vi "Get WorksheetPart.vi"(8 "error in":errorcluster, 10 "Sheet Name":string, 11 "SpreadsheetDocument in":refnum<k24>) -> (0 "error out":errorcluster, 2 "WorksheetPart":refnum<k24>, 3 "SpreadsheetDocument out":refnum<k24>)   [LabVIEW 2021, in "Open Xml.lvlib"]
uses:
  Open Xml.lvlib
  D:/git/Open-Xml-LabVIEW/dll/DocumentFormat.OpenXml.dll
  dll/DocumentFormat.OpenXml.dll
  D:/git/Open-Xml-LabVIEW/dll/DocumentFormat.OpenXml.Framework.dll
  dll/DocumentFormat.OpenXml.Framework.dll
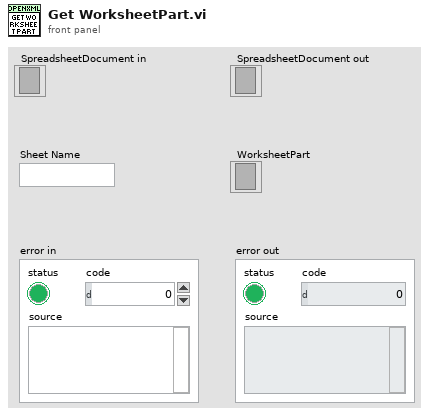
[diagram p1: front panel]
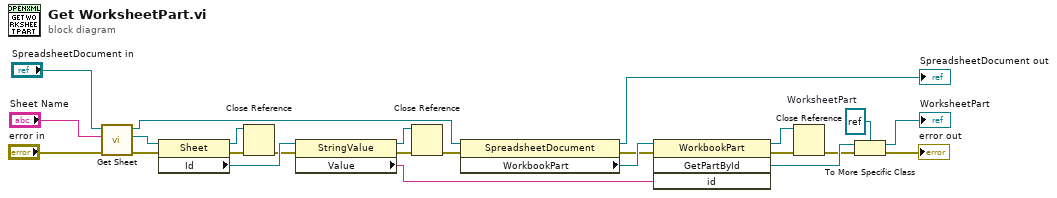
[diagram p0: block diagram]
diagram:
  w6 = refnum<k24> refnum  # WorksheetPart
  n1 = call "Get Sheet.vi"("error in"="error in", "SheetName"="Sheet Name", "SpreadsheetDoc in"="SpreadsheetDocument in") -> ("error out"=w15:errorcluster, "Sheet"=w14:refnum<k24>, "SpreadsheetDoc out"=w21:refnum<k24>)  [unwired: 6 in]
  n2 = property class="Sheet"(reference=w14, error in=w15) -> (reference out=w9:refnum<k24>, error out=w16:errorcluster, "Id"=w17:refnum<k24>)
  n3 = Close Reference(reference=w9, error in (no error)=w16) -> (error out=w10:errorcluster)
  n4 = property class="StringValue"(reference=w17, error in=w10) -> (reference out=w3:refnum<k24>, error out=w12:errorcluster, "Value"=w13:string)
  n5 = Close Reference(reference=w3, error in (no error)=w12) -> (error out=w4:errorcluster)
  n6 = property class="SpreadsheetDocument"(reference=w21, error in=w4) -> (reference out=→"SpreadsheetDocument out":refnum<k24>, error out=w19:errorcluster, "WorkbookPart"=w20:refnum<k24>)
  n7 = invoke class="WorkbookPart" method="GetPartById"(reference=w20, error in=w19, "id"=w13) -> (reference out=w1:refnum<k24>, error out=w18:errorcluster, "GetPartById"=w7:refnum<k24>)  [unwired: 1 in, 1 out]
  n8 = Close Reference(reference=w1, error in (no error)=w18) -> (error out=w2:errorcluster)
  n9 = To More Specific Class(target class=w6, reference=w7, error in=w2) -> (specific class reference=→"WorksheetPart":refnum<k24>, error out=→"error out":errorcluster)
